vi "Signal Create.vi"(8 "error in (no error)":errorcluster, 9 "Dimension":refnum<data-value>, 10 "Raw":refnum<data-value>, 11 "Data":refnum<data-value>) -> (0 "error out":errorcluster, 3 "Signal DVR out":refnum<data-value>)   [LabVIEW 2012, in "MDSplus.lvlib"]
uses:
  <vilib>/MDSplus/Library/MDSplus.lvlib
  <vilib>/MDSplus/Classes/Data_Class/Data.lvclass
  <vilib>/MDSplus/Classes/Data_Class/Compound_Class/Signal_Class/Signal.lvclass
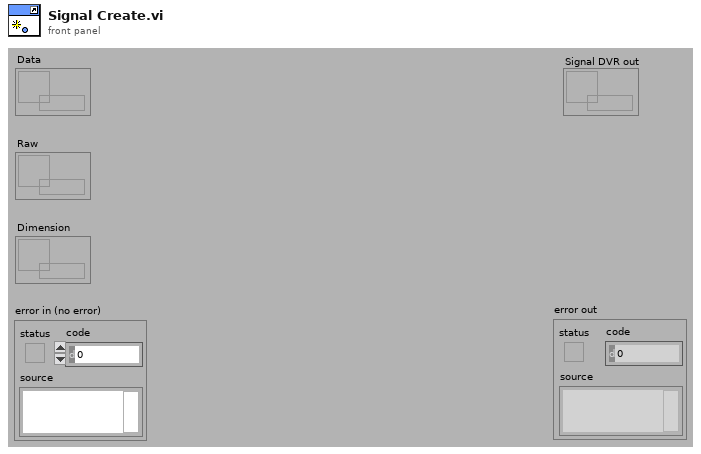
[diagram p1: front panel]
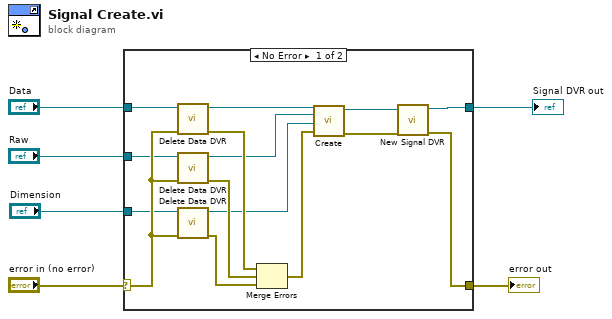
[diagram p0: block diagram]
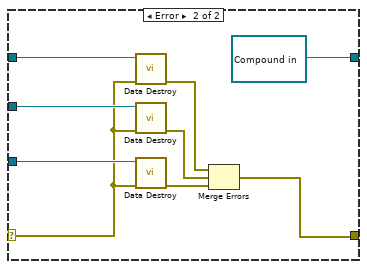
[diagram p2: hidden frame]
diagram:
  n1 = case shown="No Error" "error in (no error)" {
    selector: "error in (no error)" -> [w20 w27]
    tunnel: "Data" -> [w21 w30]
    tunnel: "Raw" -> [w19 w29]
    tunnel: "Dimension" -> [w18 w28]
    tunnel: [w14 w23] -> w2
    tunnel: [w7 refnum<data-value> refnum ("Signal DVR out")] -> w1
    frame No Error {
      n2 = call <vilib>:"Delete Data DVR.vi"("error in (no error)"=w20, "Data DVR in"=w21) -> ("error out"=w15:errorcluster, "Data out"=w13:refnum<class "Data.lvclass">)  [unwired: 8 in]
      n3 = call <vilib>:"Delete Data DVR.vi"("error in (no error)"=w20, "Data DVR in"=w19) -> ("error out"=w16:errorcluster, "Data out"=w12:refnum<class "Data.lvclass">)  [unwired: 8 in]
      n4 = call <vilib>:"Delete Data DVR.vi"("error in (no error)"=w20, "Data DVR in"=w18) -> ("error out"=w17:errorcluster, "Data out"=w11:refnum<class "Data.lvclass">)  [unwired: 8 in]
      n5 = Merge Errors(w15, w16, w17) -> (w10:errorcluster)
      n6 = call <vilib>:"Create.vi"("error in (no error)"=w10, "Dimension"=w11, "Raw"=w12, "Data"=w13) -> ("error out"=w8:errorcluster, "Signal out"=w9:refnum<class "Signal.lvclass">)  [unwired: 6 in]
      n7 = call <vilib>:"New Signal DVR.vi"("error in (no error)"=w8, "Signal in"=w9) -> ("error out"=w14:errorcluster, "Signal DVR out"=w7:refnum<data-value>)  [unwired: 8 in]
    }
    frame Error {
      n8 = call <vilib>:"Data Destroy.vi"("error in (no error)"=w27, "Data DVR in"=w30) -> ("error out"=w26:errorcluster)  [unwired: 9 in]
      n9 = call <vilib>:"Data Destroy.vi"("error in (no error)"=w27, "Data DVR in"=w29) -> ("error out"=w25:errorcluster)  [unwired: 9 in]
      n10 = call <vilib>:"Data Destroy.vi"("error in (no error)"=w27, "Data DVR in"=w28) -> ("error out"=w24:errorcluster)  [unwired: 9 in]
      n11 = Merge Errors(w26, w25, w24) -> (w23:errorcluster)
    }
  }
  "error out" <- w2
  "Signal DVR out" <- w1
